vi "LabVIEW_design.vi"() -> ()   [LabVIEW 2019]
uses:
  <vilib>/Instr/_visa.llb/VISA Configure Serial Port (Instr).vi
panel:
  out "黑名单":string[][](table)
  out "在网状态表":string[][](table)
  out "result string 11":string
  out "result string 10":string
  out "result string 9":string
  out "result string 3":string
  out "result string 4":string
  out "result string 5":string
  out "数据曲线":cluster{"横坐标":dbl[], i32[]}(graph)
  in  "设置频率":bool
  in  "Link终端地址":dbl[](array[numeric])
  in  "退网地址":dbl[](array[numeric])
  in  "入网地址":dbl[](array[numeric])
  in  "采集数据":bool
  in  "退网":bool
  in  "更新黑名单":bool
  in  "更新在网状态表":bool
  in  "入网":bool
  out "提示信息":string
  in  "信道频率":string[](array[string])
  in  "空字符串":string
  in  "result string 2":string
  in  "result string":string
  out "数据":i32
  out "read buffer":string
  in  "横坐标":dbl[](array[numeric])=[1.0, 2.0, 3.0, 4.0, 5.0, 6.0]
  in  "串口号":refnum<visa-resource-name>
  # "更新在网状态表"
  # "更新黑名单"
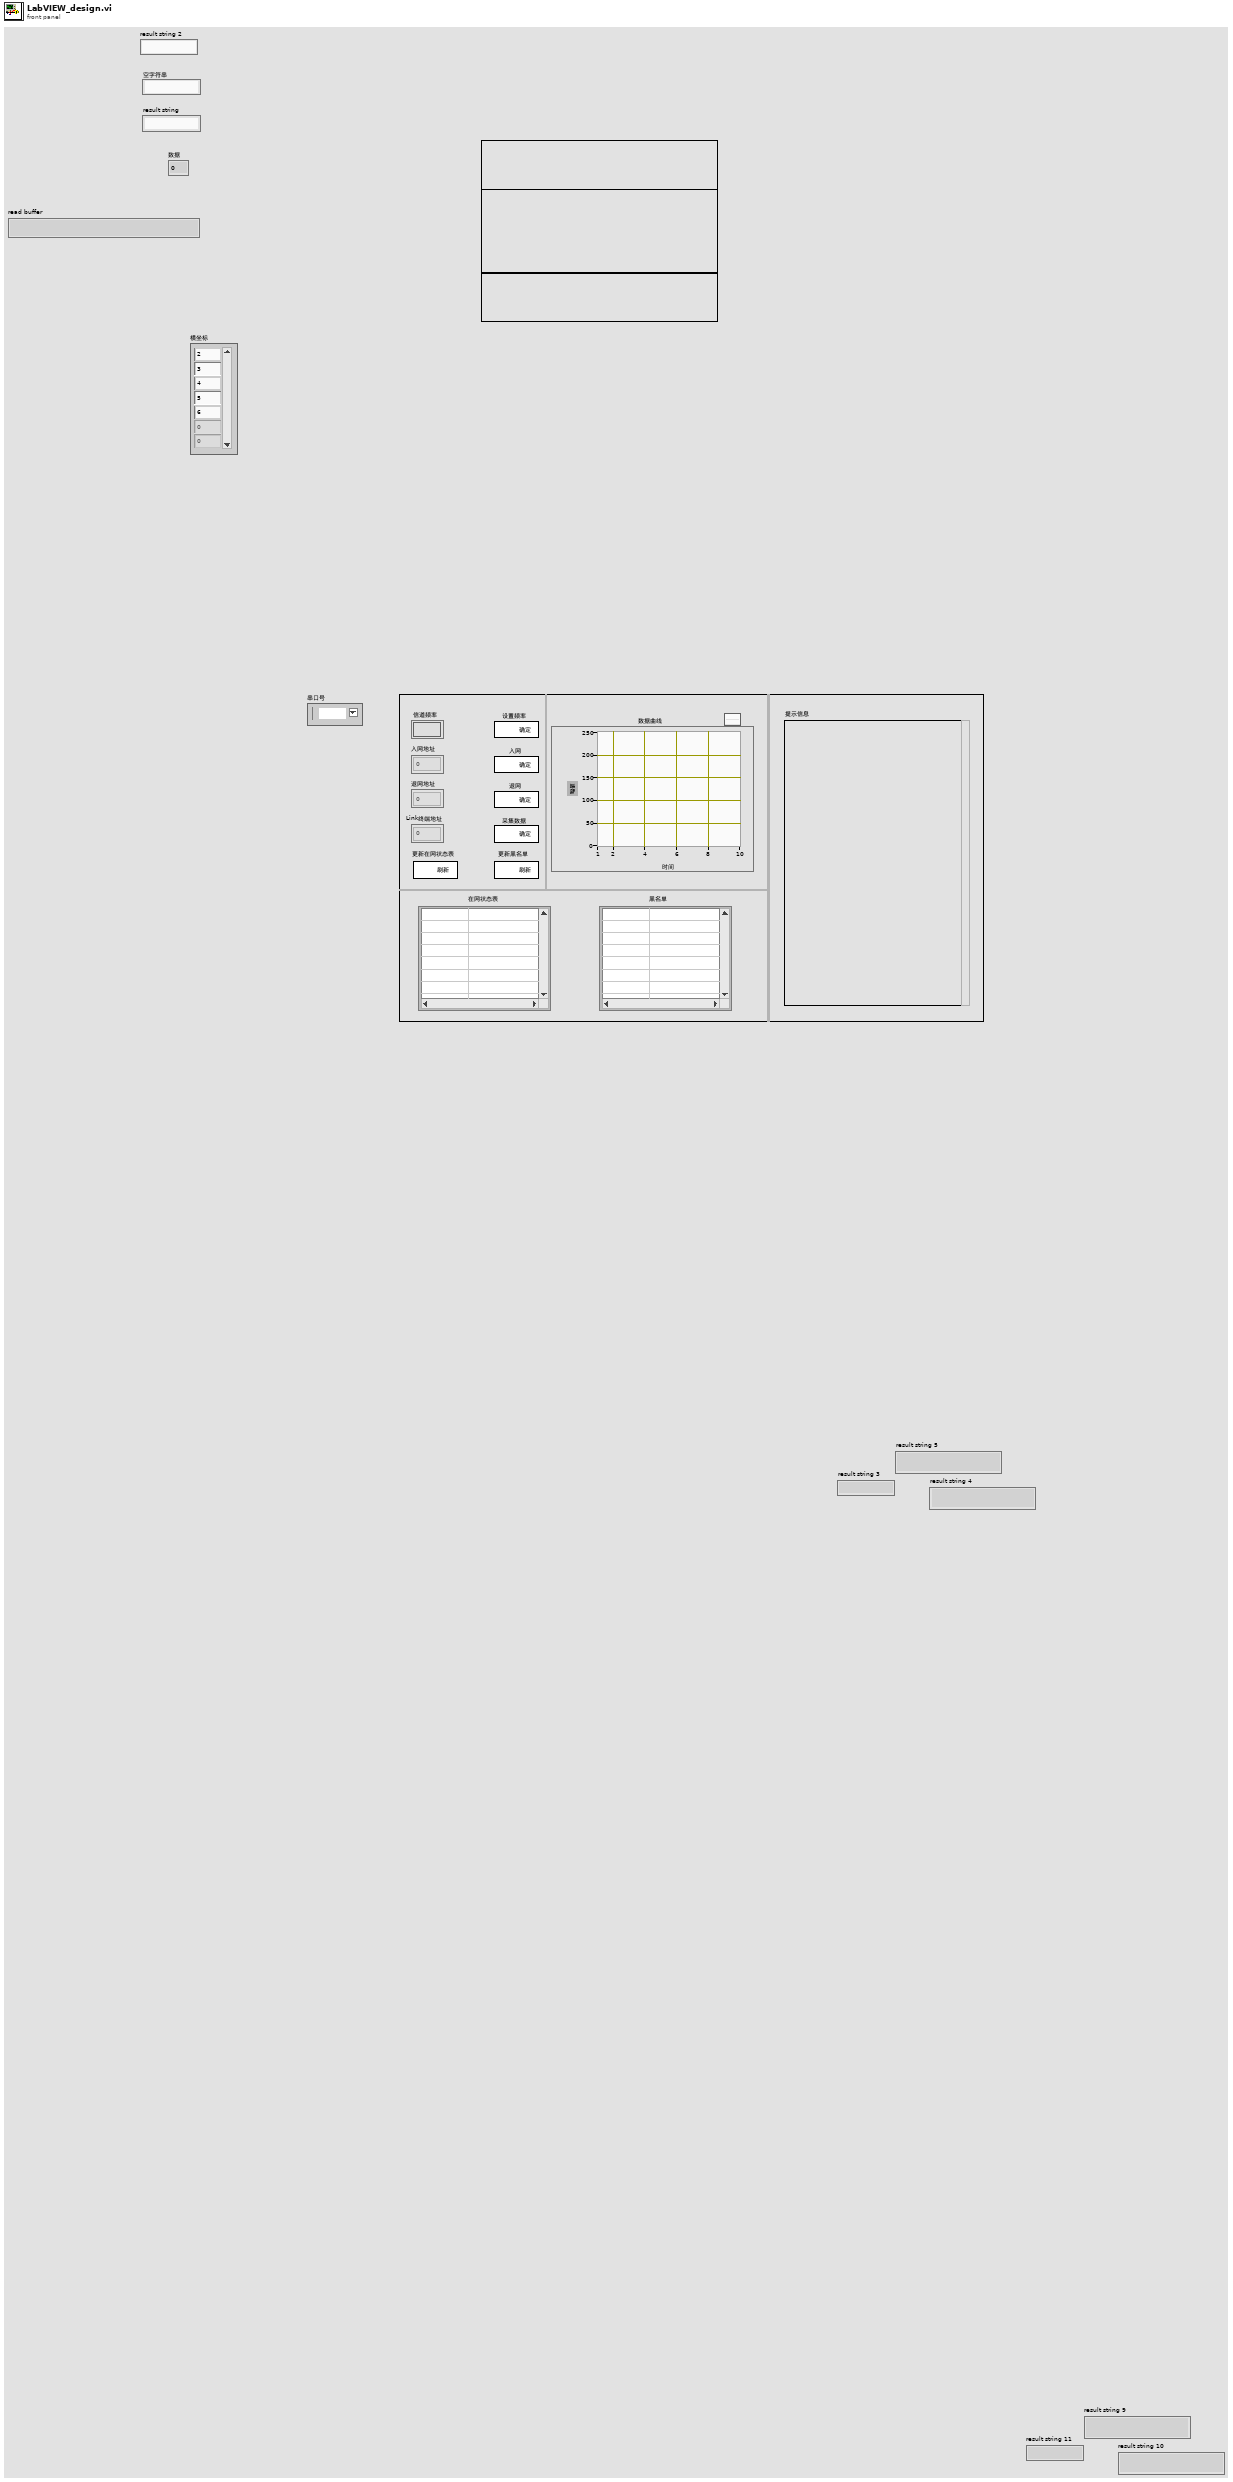
[diagram p1: front panel]
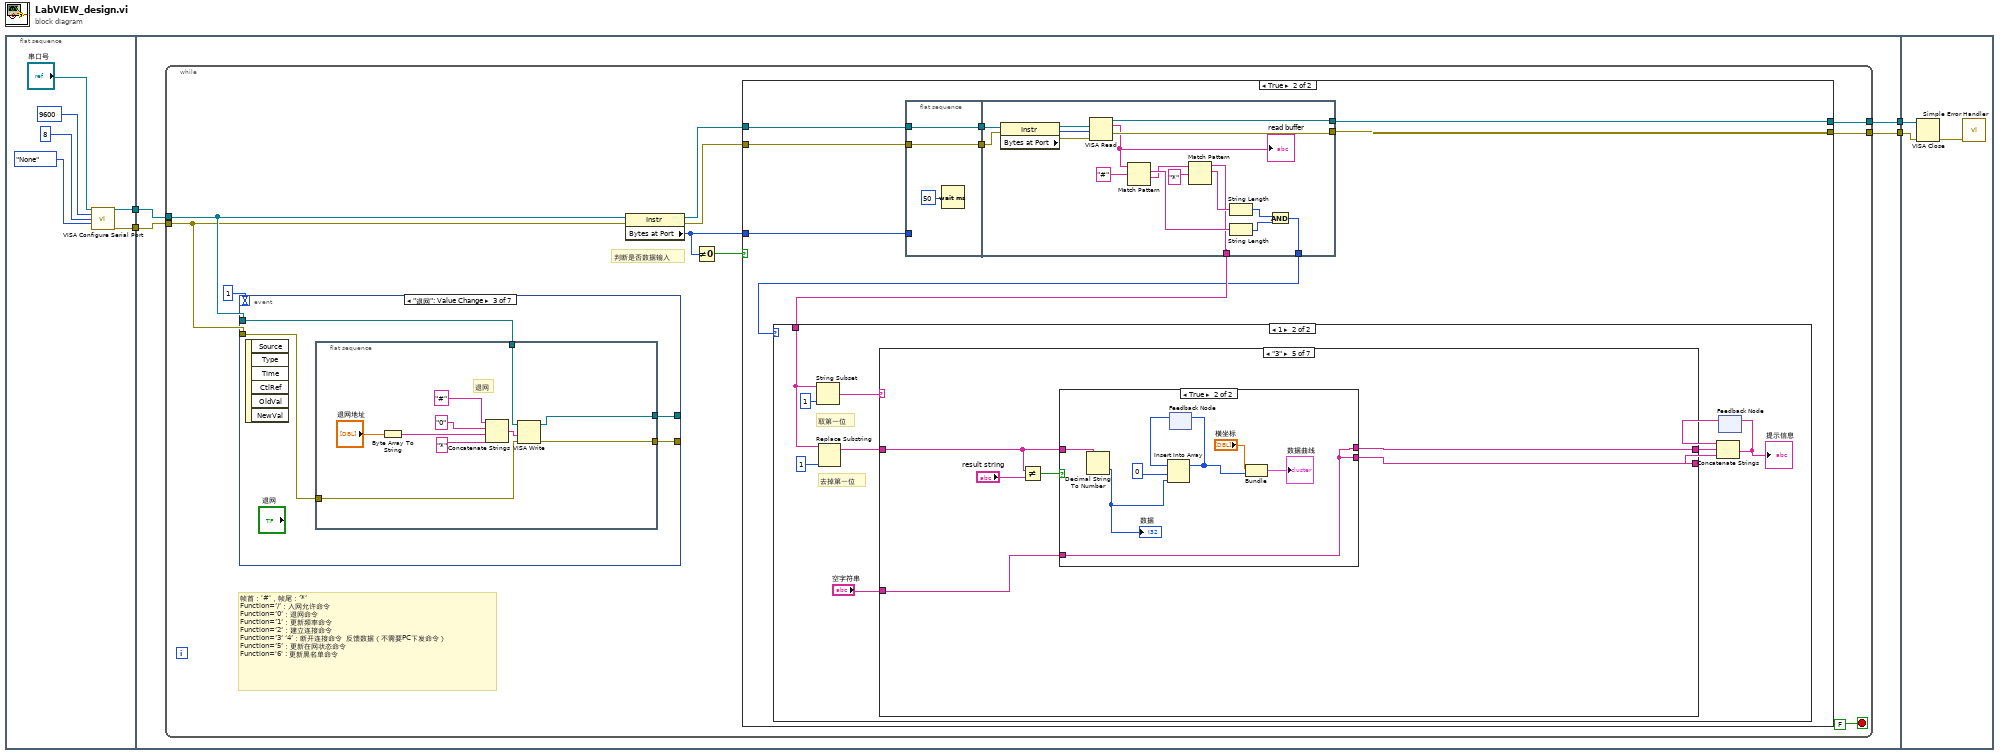
[diagram p0: block diagram]
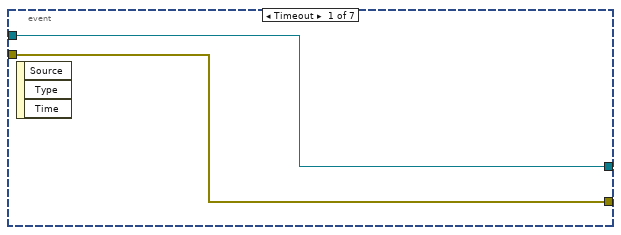
[diagram p2: hidden frame]
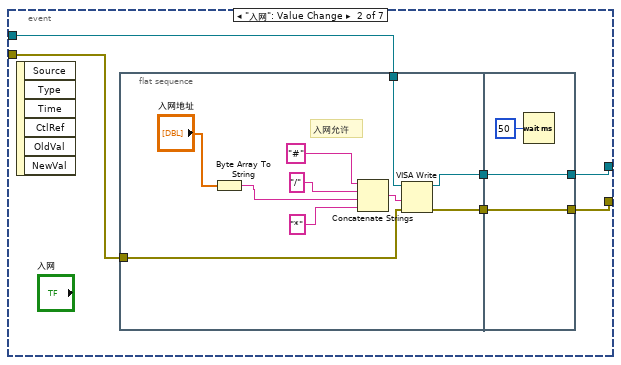
[diagram p3: hidden frame]
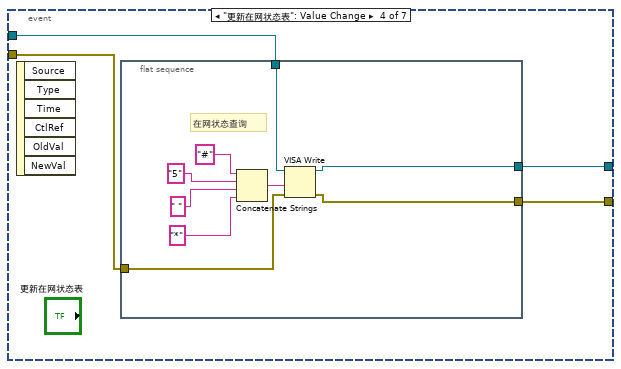
[diagram p4: hidden frame]
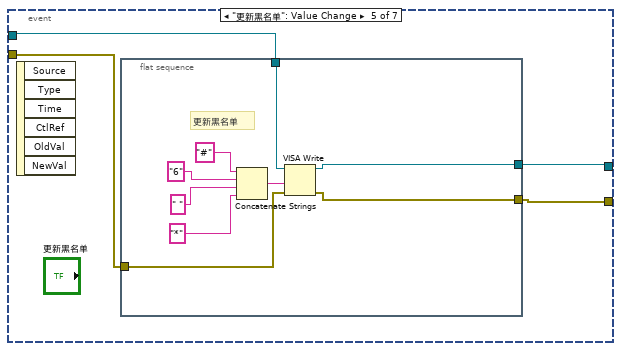
[diagram p5: hidden frame]
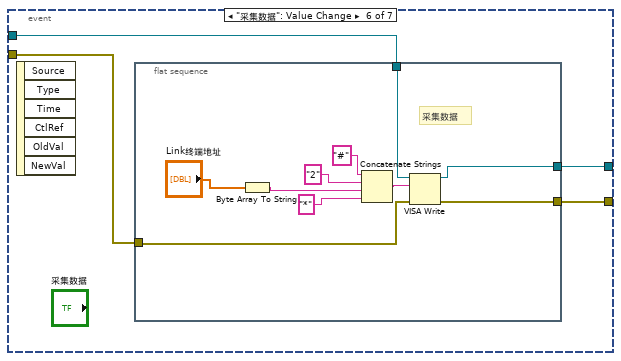
[diagram p6: hidden frame]
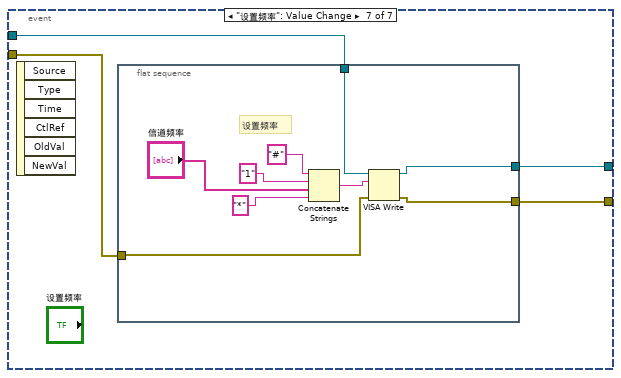
[diagram p7: hidden frame]
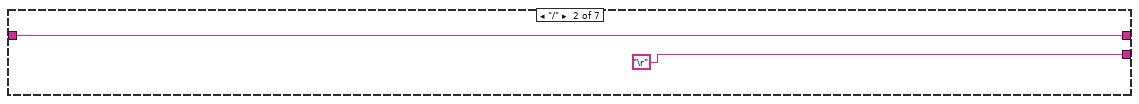
[diagram p11: hidden frame]
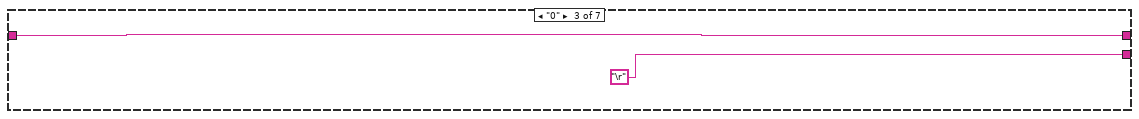
[diagram p12: hidden frame]
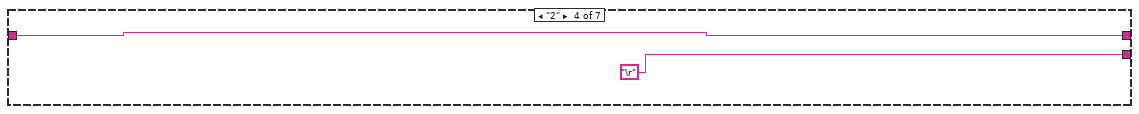
[diagram p13: hidden frame]
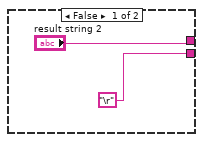
[diagram p14: hidden frame]
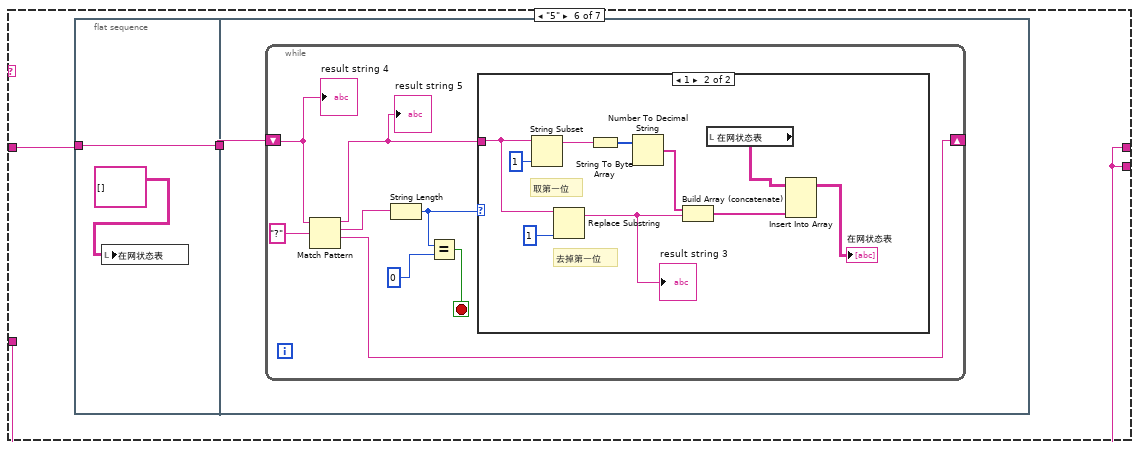
[diagram p15: hidden frame]
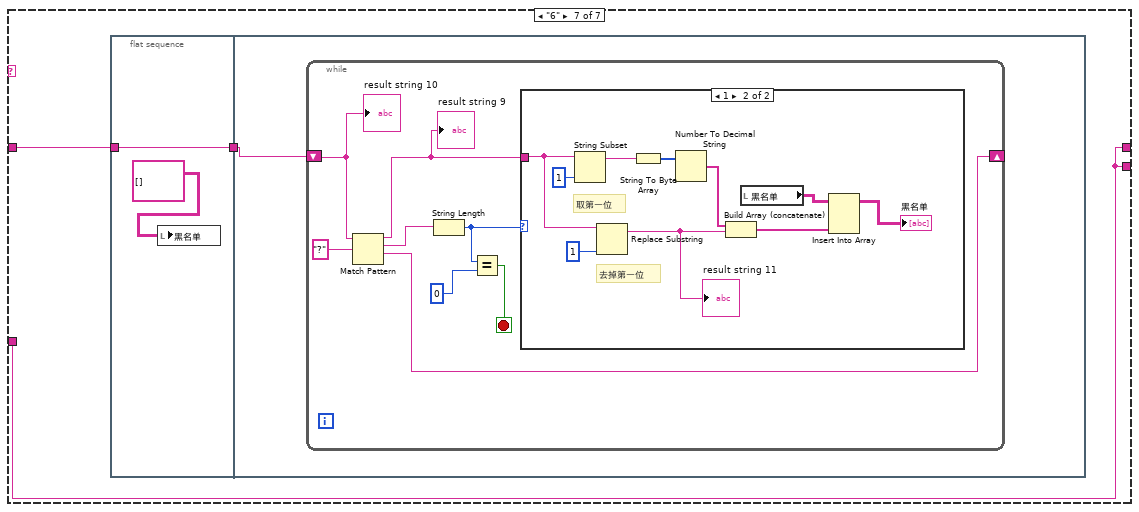
[diagram p17: hidden frame]
diagram:
  n1 = flat-sequence {
    tunnel: [w7] -> w4
    tunnel: [w6] -> w3
    tunnel: w4 -> [w14]
    tunnel: w3 -> [w13]
    tunnel: [w12] -> w2
    tunnel: [w11] -> w1
    tunnel: w2 -> [w226]
    tunnel: w1 -> [w225]
    frame #0 {
      n2 = call-poly "VISA Configure Serial Port"("VISA resource name"="串口号", "baud rate (9600)"=u32 9600, "data bits (8)"=u16 8, "parity (0:none)"=enum16{"None", "Odd", "Even", "Mark", "Space"}."None") -> ("VISA resource name out"=w6:refnum<visa-resource-name>, "error out"=w7:errorcluster)  [unwired: 10 in]
    }
    frame #1 {
      n3 = while {
        tunnel: w14 -> [w15]
        tunnel: w13 -> [w16]
        tunnel: [w22] -> w12
        tunnel: [w23] -> w11
        stop <- FALSE stop-if-true
        # "帧首：'#'，帧尾：’*‘\nFunction=’/‘：入网允许命令\nFunction=’0‘：退网命令\nFunction=’1‘：更新频率命令\nFunction=’2‘：建立连接命令\nFunction=’3‘ ‘4’：断开连接命令  反馈数据（不需要PC下发命令）\nFunction=’5‘：更新在网状态命令\nFunction='6' : 更新黑名单命令"
        # "判断是否数据输入"
        n4 = event shown="[2] \"退网\": Value Change" {
          selector: _ -> [_ _ _ _ _ _ _]
          dyn-events: _ -> [_ _ _ _ _ _ _]
          timeout: 1 -> [_ _ _ _ _ _ _]
          tunnel: w16 -> [w26 w31 w49 w63 w75 w89 w103]
          tunnel: w15 -> [w25 w32 w48 w62 w76 w88 w102]
          tunnel: [w26 w30 w47 w61 w74 w87 w101] -> _
          tunnel: [w25 w29 w46 w60 w73 w86 w100] -> _
          event Timeout {
            n5 = event-data() -> ()  [unwired: 1 in, 3 out]
          }
          event "入网": Value Change {
            n6 = event-data() -> ()  [unwired: 1 in, 6 out]
            n7 = flat-sequence {
              tunnel: w31 -> [w38]
              tunnel: w32 -> [w35]
              tunnel: [w37] -> w28
              tunnel: [w36] -> w27
              tunnel: [w44] -> w29
              tunnel: [w45] -> w30
              tunnel: w28 -> [w45]
              tunnel: w27 -> [w44]
              frame #0 {
                # "入网允许"
                n8 = Byte Array To String(unsigned byte array="入网地址") -> (string=w34:string)
                n9 = Concatenate Strings("#" ("字符串"), "/" ("字符串"), w34, "*" ("字符串")) -> (w42:string)
                n10 = VISA Write(VISA resource name=w38, write buffer=w42, error in (no error)=w35) -> (VISA resource name out=w37:refnum<visa-resource-name>, error out=w36:errorcluster)  [unwired: 1 out]
              }
              frame #1 {
                n11 = Wait (ms)(milliseconds to wait=u32 50 ("等待时间（毫秒）")) -> ()  [unwired: 1 out]
              }
            }
          }
          event "退网": Value Change {
            n12 = event-data() -> ()  [unwired: 1 in, 6 out]
            n13 = flat-sequence {
              tunnel: w49 -> [w55]
              tunnel: w48 -> [w54]
              tunnel: [w53] -> w47
              tunnel: [w52] -> w46
              frame #0 {
                # "退网"
                n14 = Byte Array To String(unsigned byte array="退网地址") -> (string=w51:string)
                n15 = Concatenate Strings("#" ("字符串"), "0" ("字符串"), w51, "*" ("字符串")) -> (w59:string)
                n16 = VISA Write(VISA resource name=w55, write buffer=w59, error in (no error)=w54) -> (VISA resource name out=w53:refnum<visa-resource-name>, error out=w52:errorcluster)  [unwired: 1 out]
              }
            }
          }
          event "更新在网状态表": Value Change {
            n17 = event-data() -> ()  [unwired: 1 in, 6 out]
            n18 = flat-sequence {
              tunnel: w63 -> [w66]
              tunnel: w62 -> [w69]
              tunnel: [w68] -> w61
              tunnel: [w67] -> w60
              frame #0 {
                # "在网状态查询"
                n19 = Concatenate Strings("#" ("字符串"), "5" ("字符串"), " " ("字符串"), "*" ("字符串")) -> (w72:string)
                n20 = VISA Write(VISA resource name=w66, write buffer=w72, error in (no error)=w69) -> (VISA resource name out=w68:refnum<visa-resource-name>, error out=w67:errorcluster)  [unwired: 1 out]
              }
            }
          }
          event "更新黑名单": Value Change {
            n21 = event-data() -> ()  [unwired: 1 in, 6 out]
            n22 = flat-sequence {
              tunnel: w75 -> [w79]
              tunnel: w76 -> [w82]
              tunnel: [w81] -> w74
              tunnel: [w80] -> w73
              frame #0 {
                # "更新黑名单"
                n23 = Concatenate Strings("#" ("字符串"), "6" ("字符串"), " " ("字符串"), "*" ("字符串")) -> (w85:string)
                n24 = VISA Write(VISA resource name=w79, write buffer=w85, error in (no error)=w82) -> (VISA resource name out=w81:refnum<visa-resource-name>, error out=w80:errorcluster)  [unwired: 1 out]
              }
            }
          }
          event "采集数据": Value Change {
            n25 = event-data() -> ()  [unwired: 1 in, 6 out]
            n26 = flat-sequence {
              tunnel: w89 -> [w95]
              tunnel: w88 -> [w94]
              tunnel: [w93] -> w87
              tunnel: [w92] -> w86
              frame #0 {
                # "采集数据"
                n27 = Byte Array To String(unsigned byte array="Link终端地址") -> (string=w91:string)
                n28 = Concatenate Strings("#" ("字符串"), "2" ("字符串"), w91, "*" ("字符串")) -> (w99:string)
                n29 = VISA Write(VISA resource name=w95, write buffer=w99, error in (no error)=w94) -> (VISA resource name out=w93:refnum<visa-resource-name>, error out=w92:errorcluster)  [unwired: 1 out]
              }
            }
          }
          event "设置频率": Value Change {
            n30 = event-data() -> ()  [unwired: 1 in, 6 out]
            n31 = flat-sequence {
              tunnel: w103 -> [w108]
              tunnel: w102 -> [w107]
              tunnel: [w106] -> w101
              tunnel: [w105] -> w100
              frame #0 {
                # "设置频率"
                n32 = Concatenate Strings("#" ("字符串"), "1" ("字符串"), "信道频率", "*" ("字符串")) -> (w109:string)
                n33 = VISA Write(VISA resource name=w108, write buffer=w109, error in (no error)=w107) -> (VISA resource name out=w106:refnum<visa-resource-name>, error out=w105:errorcluster)  [unwired: 1 out]
              }
            }
          }
        }
        n34 = property class="Instr"(reference=w16, error in=w15) -> (reference out=w21:refnum<visa-resource-name>, error out=w19:errorcluster, "Bytes at Port"=w20:u32)
        n35 = Not Equal To 0?(x=w20) -> (x != 0?=w24:bool)
        n36 = case shown="True" w24 {
          tunnel: w19 -> [w113 w121]
          tunnel: w21 -> [w114 w123]
          tunnel: [w114 w122] -> w23
          tunnel: [w113 w120] -> w22
          tunnel: w20 -> [_ w119]
          frame False {
          }
          frame True {
            n37 = case shown="1" w115 {
              tunnel: w116 -> [_ w150]
              frame 0, Default {
              }
              frame 1 {
                # "去掉第一位"
                # "取第一位"
                n38 = String Subset ("截取字符串")(string=w150, length (rest)=1 ("length (rest)")) -> (substring=w152:string)  [unwired: 1 in]
                n39 = Replace Substring(2:1 ("length (rest)"), 5:w150) -> (1:w149:string)  [unwired: 2 in, 1 out]
                n40 = case shown="\"3\"" w152 {
                  tunnel: w149 -> [_ w156 w158 w160 w164 w179 w203]
                  tunnel: [w154 w156 w158 w160 w163 w178 w202] -> w147
                  tunnel: [w154 "\r" "\r" "\r" w162 w178 w202] -> w146
                  tunnel: "空字符串" -> [w154 _ _ _ w161 w178 w202]
                  frame " ", Default {
                  }
                  frame "/" {
                  }
                  frame "0" {
                  }
                  frame "2" {
                  }
                  frame "3" {
                    n41 = Not Equal?(x=w164, y="result string") -> (x != y?=w165:bool)
                    n42 = case shown="True" w165 {
                      tunnel: w164 -> [_ w173]
                      tunnel: ["result string 2" w170] -> w163
                      tunnel: ["\r" w170] -> w162
                      tunnel: w161 -> [_ w170]
                      frame False {
                      }
                      frame True {
                        n43 = Decimal String To Number(string=w173) -> (number=w172:i32)  [unwired: 2 in, 1 out]
                        "数据" <- w172
                        n44 = feedback #1() -> (w176:i32[])  [unwired: 1 in]
                        n45 = Insert Into Array(array=w176, index=0, new element=w172) -> (w174:i32[])
                        n46 = feedback-in #1(w174) -> ()
                        n47 = Bundle("横坐标"="横坐标", w174) -> (→"数据曲线":cluster{"横坐标":dbl[], i32[]})  [unwired: 1 in]
                      }
                    }
                  }
                  frame "5" {
                    n48 = flat-sequence {
                      tunnel: w179 -> [w181]
                      tunnel: [w181] -> w177
                      tunnel: w177 -> [w182]
                      frame #0 {
                        n49 = local write "在网状态表"(string[][] [] ("表格控件 3")) -> ()
                      }
                      frame #1 {
                        n50 = while {
                          shift-right: [w186] -> _
                          shift-left: w182 -> [w184]
                          stop <- w188 stop-if-true
                          n51 = Match Pattern(string=w184, regular expression="?") -> (before substring=w183:string, match substring=w185:string, after substring=w186:string)  [unwired: 1 in, 1 out]
                          "result string 5" <- w183
                          n52 = String Length(string=w185) -> (length=w189:i32)
                          n53 = Equal?(x=w189, y=0) -> (x = y?=w188:bool)
                          n54 = case shown="1" w189 {
                            tunnel: w183 -> [_ w196]
                            frame 0, Default {
                            }
                            frame 1 {
                              # "去掉第一位"
                              # "取第一位"
                              n55 = String Subset ("截取字符串")(string=w196, length (rest)=1 ("length (rest)")) -> (substring=w199:string)  [unwired: 1 in]
                              n56 = Replace Substring(2:1 ("length (rest)"), 5:w196) -> (1:w195:string)  [unwired: 2 in, 1 out]
                              "result string 3" <- w195
                              n57 = String To Byte Array(string=w199) -> (unsigned byte array=w198:u8[])
                              n58 = Number To Decimal String(number=w198) -> (decimal integer string=w194:string[])  [unwired: 1 in]
                              n59 = Build Array (concatenate)(w194, w195) -> (w193:string[])
                              n60 = local read "在网状态表"() -> (w192:string[][])
                              n61 = Insert Into Array(array=w192, new element=w193) -> (→"在网状态表":string[][])  [unwired: 2 in]
                            }
                          }
                          "result string 4" <- w184
                        }
                      }
                    }
                  }
                  frame "6" {
                    n62 = flat-sequence {
                      tunnel: w203 -> [w205]
                      tunnel: [w205] -> w201
                      tunnel: w201 -> [w206]
                      frame #0 {
                        n63 = local write "黑名单"(string[][] [] ("表格控件 3")) -> ()
                      }
                      frame #1 {
                        n64 = while {
                          shift-right: [w210] -> _
                          shift-left: w206 -> [w208]
                          stop <- w212 stop-if-true
                          n65 = Match Pattern(string=w208, regular expression="?") -> (before substring=w207:string, match substring=w209:string, after substring=w210:string)  [unwired: 1 in, 1 out]
                          "result string 9" <- w207
                          n66 = String Length(string=w209) -> (length=w213:i32)
                          n67 = Equal?(x=w213, y=0) -> (x = y?=w212:bool)
                          n68 = case shown="1" w213 {
                            tunnel: w207 -> [_ w220]
                            frame 0, Default {
                            }
                            frame 1 {
                              # "去掉第一位"
                              # "取第一位"
                              n69 = String Subset ("截取字符串")(string=w220, length (rest)=1 ("length (rest)")) -> (substring=w223:string)  [unwired: 1 in]
                              n70 = Replace Substring(2:1 ("length (rest)"), 5:w220) -> (1:w219:string)  [unwired: 2 in, 1 out]
                              "result string 11" <- w219
                              n71 = String To Byte Array(string=w223) -> (unsigned byte array=w222:u8[])
                              n72 = Number To Decimal String(number=w222) -> (decimal integer string=w218:string[])  [unwired: 1 in]
                              n73 = Build Array (concatenate)(w218, w219) -> (w216:string[])
                              n74 = local read "黑名单"() -> (w217:string[][])
                              n75 = Insert Into Array(array=w217, new element=w216) -> (→"黑名单":string[][])  [unwired: 2 in]
                            }
                          }
                          "result string 10" <- w208
                        }
                      }
                    }
                  }
                }
                n76 = feedback #2() -> (w148:string)  [unwired: 1 in]
                n77 = Concatenate Strings(w148, w147, w146) -> (w144:string)
                "提示信息" <- w144
                n78 = feedback-in #2(w144) -> ()
              }
            }
            n79 = flat-sequence {
              tunnel: w119 -> [_]
              tunnel: w121 -> [w125]
              tunnel: w123 -> [w126]
              tunnel: [w126] -> w118
              tunnel: [w125] -> w117
              tunnel: [w143] -> w122
              tunnel: [w142] -> w120
              tunnel: [w134] -> w115
              tunnel: w118 -> [w132]
              tunnel: w117 -> [w131]
              tunnel: [w127] -> w116
              frame #0 {
                n80 = Wait (ms)(milliseconds to wait=u32 50 ("等待时间（毫秒）")) -> ()  [unwired: 1 out]
              }
              frame #1 {
                n81 = property class="Instr"(reference=w132, error in=w131) -> (reference out=w129:refnum<visa-resource-name>, error out=w128:errorcluster, "Bytes at Port"=w130:u32)
                n82 = VISA Read(VISA resource name=w129, byte count=w130, error in (no error)=w128) -> (VISA resource name out=w143:refnum<visa-resource-name>, read buffer=w141:string, error out=w142:errorcluster)  [unwired: 1 out]
                "read buffer" <- w141
                n83 = Match Pattern(string=w141, regular expression="#") -> (match substring=w138:string, after substring=w133:string)  [unwired: 1 in, 2 out]
                n84 = Match Pattern(string=w133, regular expression="*") -> (before substring=w127:string, match substring=w137:string)  [unwired: 1 in, 2 out]
                n85 = String Length(string=w137) -> (length=w135:i32)
                n86 = String Length(string=w138) -> (length=w136:i32)
                n87 = And(x=w135, y=w136) -> (x .and. y?=w134:i32)
              }
            }
          }
        }
      }
    }
    frame #2 {
      n88 = VISA Close(VISA resource name=w225, error in (no error)=w226) -> (error out=w227:errorcluster)
      n89 = call <vilib>:"Simple Error Handler.vi"("error in (no error)"=w227) -> ()  [unwired: 4 in, 5 out]
    }
  }
